vi "SyncSum.vi"(8 "error in (no error)":errorcluster, 10 "B":i32, 11 "A":i32) -> (0 "error out":errorcluster, 3 "Sum":i32)   [LabVIEW 2016, in "DemoSkeleton.lvlib"]
uses:
  DemoSkeleton.lvlib
  skeleton_lv_event_lvrt.dll
  skeleton_lv_event_lv.dll
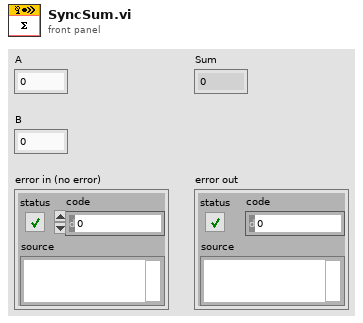
[diagram p1: front panel]
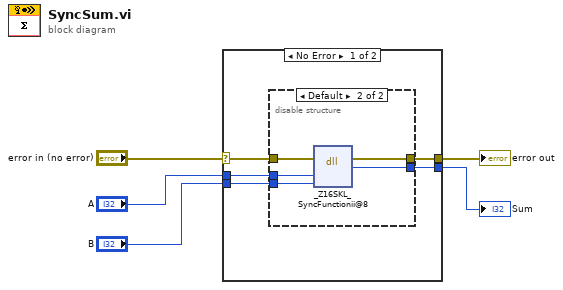
[diagram p0: block diagram]
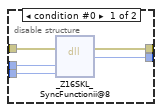
[diagram p2: hidden frame]
diagram:
  n1 = case shown="No Error" "error in (no error)" {
    selector: "error in (no error)" -> [w10 w21]
    tunnel: "A" -> [w9 _]
    tunnel: "B" -> [w8 _]
    tunnel: [w7 _] -> w2
    tunnel: [w6 w21] -> w1
    frame No Error {
      n2 = disable-structure shown="Default" {
        disable-tunnel: [w13 w19] -> w7
        disable-tunnel: w10 -> [w15 w16]
        disable-tunnel: [w14 w20] -> w6
        disable-tunnel: w9 -> [w12 w18]
        disable-tunnel: w8 -> [w11 w17]
        frame condition #0 {
          n3 = dll-call lib="C:/Users/loic.wohleber/Desktop/PostLvUserEvent_Demo/Sources/LabVIEW/Library/DemoSkeleton/skeleton_lv_event_lvrt.dll" fn="_Z16SKL_SyncFunctionii@8" label="SyncSum_RT"(error in=w15, "A"=w12, "B"=w11) -> (error out=w14:errorcluster, "Sum"=w13:i32)  [unwired: 4 in, 1 out]
        }
        frame condition #1 (active) {
          n4 = dll-call lib="C:/Users/loic.wohleber/Desktop/PostLvUserEvent_Demo/Sources/LabVIEW/Library/DemoSkeleton/skeleton_lv_event_lv.dll" fn="_Z16SKL_SyncFunctionii@8" label="SyncSum"(error in=w16, "A"=w18, "B"=w17) -> (error out=w20:errorcluster, "Sum"=w19:i32)  [unwired: 4 in, 1 out]
        }
      }
    }
    frame Error {
    }
  }
  "Sum" <- w2
  "error out" <- w1
